vi "00T_CreateLOGfile.vi"(11 "LOG file":path) -> (3 "refnum out":refnum<file>)   [LabVIEW 2017]
uses:
  <vilib>/Utility/error.llb/whitespace.ctl
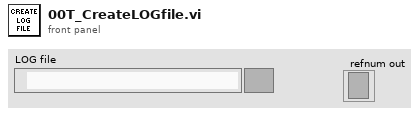
[diagram p1: front panel]
types:
  T1 = typedef "whitespace.ctl" = u16
  T2 = enum16{"open", "replace", "create", "open or create", "replace or create", "replace or create with confirmation"}
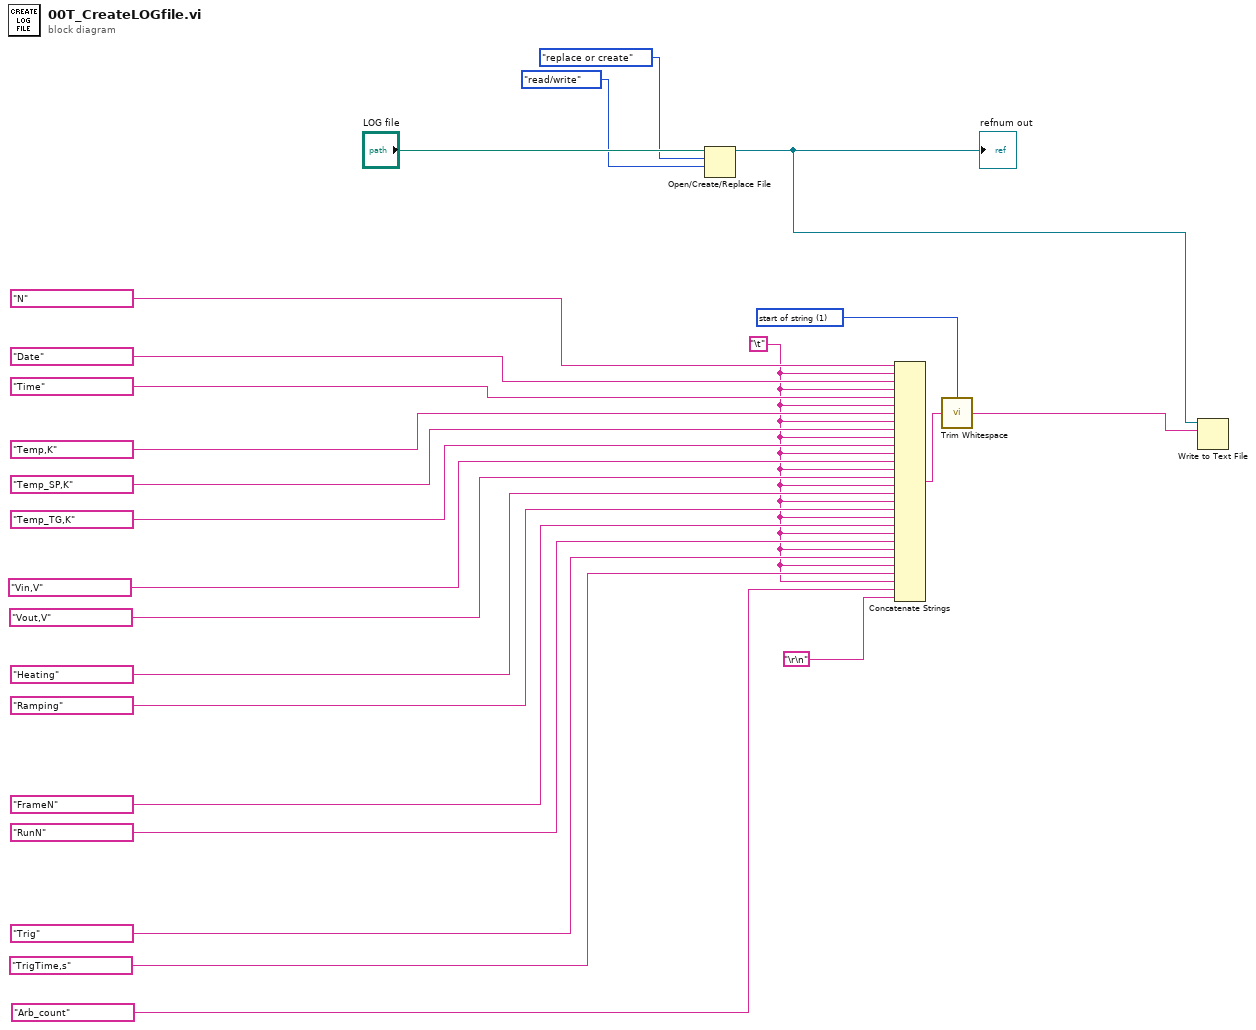
[diagram p0: block diagram]
diagram:
  w3 = "\t"
  w20 = T1 1 items=["both", "start of string", "end of string"] ("location (both)")
  n1 = Open/Create/Replace File(file path (use dialog)="LOG file", operation (0:open)=T2."replace or create", access (0:read/write)=enum16{"read/write", "read-only", "write-only"}."read/write") -> (refnum out=w6:refnum<file>)  [unwired: 3 in, 2 out]
  "refnum out" <- w6
  n2 = Concatenate Strings("N" ("string"), w3, "Date" ("string"), w3, "Time" ("string"), w3, "Temp,K" ("string"), w3, "Temp_SP,K" ("string"), w3, "Temp_TG,K" ("string"), w3, "Vin,V" ("string"), w3, "Vout,V" ("string"), w3, "Heating" ("string"), w3, "Ramping" ("string"), w3, "FrameN" ("string"), w3, "RunN" ("string"), w3, "Trig" ("string"), w3, "TrigTime,s" ("string"), w3, "Arb_count" ("string"), "\r\n") -> (w21:string)
  n3 = call <vilib>:"Trim Whitespace.vi"("string"=w21, "location (both)"=w20) -> ("trimmed string"=w5:string)
  n4 = Write to Text File(file (use dialog)=w6, text=w5) -> ()  [unwired: 2 in, 3 out]
